vi "SubVI_Spatial_Mean.vi"(6 "Channel_select":i32[](array[numeric])=[1, 2, 3], 8 "error in (no error)":errorcluster, 9 "Window Size":i32, 10 "Time Array":dbl[][](array[numeric]), 11 "Downsampled EEG In":T2) -> (0 "error out":errorcluster, 3 "Spatial Mean Out":T1)   [LabVIEW 2020]
uses:
  <extravilib>/ChannelInstances/Stream-a[.](dbl)/)Channel.ctl
  <extravilib>/ChannelInstances/Stream-a[.,.](dbl)/)Channel.ctl
  <vilib>/Analysis/baseanly.llb/Mean (DBL).vi
  <extravilib>/ChannelInstances/Stream-a[.](dbl)/EndpointRead.vi
  <extravilib>/ChannelInstances/Stream-a[.,.](dbl)/Endpoint.vi
  <extravilib>/ChannelInstances/Stream-a[.](dbl)/)Channel.vi
  <resource>/ChannelSupport/_ChannelSupport/WaitIfNeeded.vi
  <extravilib>/ChannelInstances/Stream-a[.,.](dbl)/)Channel.vi
  <extravilib>/ChannelInstances/Stream-a[.](dbl).lvlib
  <vilib>/Analysis/NI_AALBase.lvlib
  <extravilib>/ChannelInstances/Stream-a[.,.](dbl).lvlib
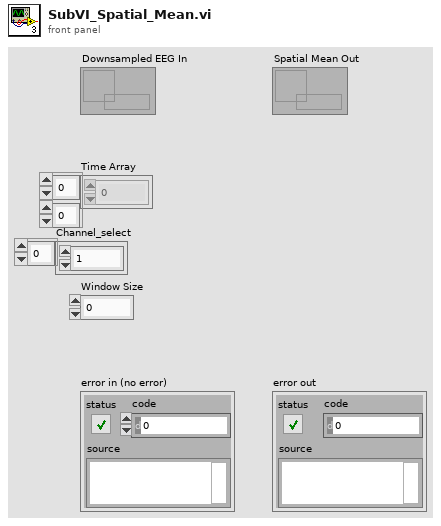
[diagram p1: front panel]
types:
  T1 = typedef "Stream-a[.,.](dbl).lvlib/)Channel.ctl" = refnum<queue>
  T2 = typedef "Stream-a[.](dbl).lvlib/)Channel.ctl" = refnum<queue>
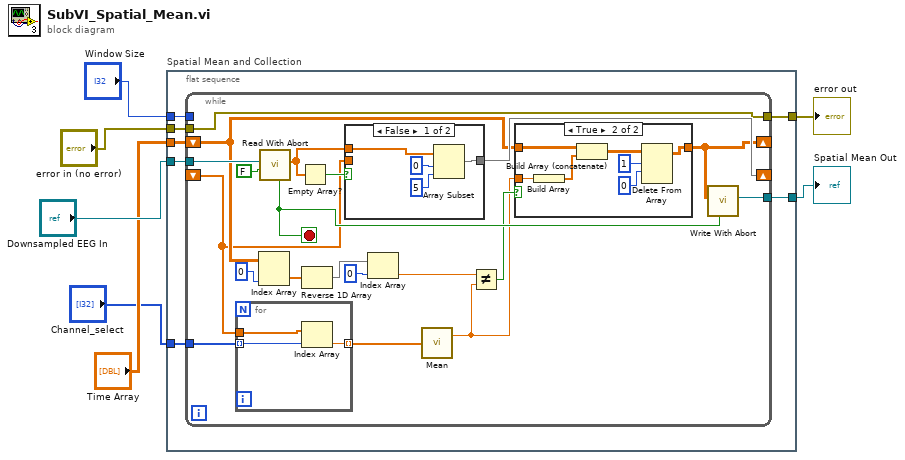
[diagram p0: block diagram]
diagram:
  n1 = flat-sequence "Spatial Mean and Collection" {
    tunnel: "Window Size" -> [w14]
    tunnel: [w13] -> w3
    tunnel: "Time Array" -> [w12]
    tunnel: "Downsampled EEG In" -> [w11]
    tunnel: [w10] -> w6
    tunnel: "error in (no error)" -> [w9]
    tunnel: "Channel_select" -> [w8]
    frame #0 {
      n2 = while {
        tunnel: w11 -> [w34]
        shift-right: [w18] -> _
        shift-left: w12 -> [w25]
        tunnel: w14 -> [_]
        tunnel: [w31] -> w13
        shift-right: [w28] -> _
        shift-left: _ -> [w17]
        tunnel: w9 -> [w27]
        tunnel: [w27] -> w10
        tunnel: w8 -> [w16]
        stop <- w32 stop-if-true
        n3 = for {
          tunnel: w17 -> [w36]
          tunnel: w16 -> [w37] mode=indexing
          tunnel: [w35] -> w15 mode=indexing
          n4 = Index Array(array=w36, index=w37) -> (element=w35:dbl)
        }
        n5 = Index Array(array=w25, index (col)=0 ("disabled index (row)")) -> (element=w23:dbl[])  [unwired: 1 in]
        n6 = call <extravilib>:"Read With Abort.vi"("abort"=FALSE, "channel"=w34) -> ("element"=w29:dbl[], "aborted?"=w32:bool)  [unwired: 4 in, 4 out]
        n7 = Empty Array?(array=w29) -> (empty?=w30:bool)
        n8 = Reverse 1D Array(array=w23) -> (reversed array=w21:dbl[])
        n9 = case shown="False" w30 {
          tunnel: w29 -> [w49 _]
          tunnel: [w46 w50] -> w28
          tunnel: w17 -> [_ w50]
          frame False {
            n10 = Array Subset(array=w49, index=0, length=5) -> (w46:dbl[])
          }
          frame True {
          }
        }
        n11 = Index Array(array=w21, index=0 ("disabled index (row)")) -> (element=w20:dbl)
        n12 = call-poly <vilib>:"Mean.vi"("X"=w15) -> ("mean"=w24:dbl)  [unwired: 1 out]
        n13 = Not Equal?(x=w20, y=w24) -> (x != y?=w26:bool)
        n14 = case shown="True" w26 {
          tunnel: w25 -> [w38 w43]
          tunnel: w24 -> [_ w44]
          tunnel: [w38 w39] -> w18
          frame False {
          }
          frame True {
            n15 = Build Array(w44) -> (w45:dbl[])
            n16 = Build Array (concatenate)(w43, w45) -> (w42:dbl[][])
            n17 = Delete From Array(array=w42, length=1, index (row)=0) -> (array with subset deleted=w39:dbl[][])  [unwired: 1 in, 1 out]
          }
        }
        n18 = call <extravilib>:"Write With Abort.vi"("abort"=w32, "element"=w18) -> ("channel"=w31:T1)  [unwired: 6 in, 3 out]
      }
    }
  }
  "error out" <- w6
  "Spatial Mean Out" <- w3
